vi "KB-CalRoi_Inner.vi"(10 "Inner ROI Descriptor (Inner Find Circular Edge 2)":T2={"Global Rectangle"=[775, 498, 995, 717], "Contours"=[{"ID"=enum."External", "Type"=7, "Coordinates"=[884, 607, 51, 109, 0, 0]}]} {"Contours"."Type" items=["No Selection", "Point", "Line", "Rectangle", "Oval", "Polygon", "Freehand Region", "Annulus", "Unused2", "Unused3", "Broken Line", "Freehand Line", "Rotated Rectangle"]}, 11 "Fitted Circle (Otter-Find Circular Edge)":T4 {"Average SNR (dB)" format="%.2f"; "Average Strength" format="%.2f"; "Roundness (Real-World)" format="%.2f"; "Radius (Real-World)" format="%.2f"; "Center (Real-World)"."Y" format="%.2f"; "Center (Real-World)"."X" format="%.2f"; "Radius (Pixels)" format="%.2f"; "Center (Pixels)"."Y" format="%.2f"; "Center (Pixels)"."X" format="%.2f"}) -> (0 "Roi":T1, 3 "New Inneer ROI":T2)   [LabVIEW 2015]
panel:
  out "Global Rectangle":i32[](array[numeric])
  out "元素":T3
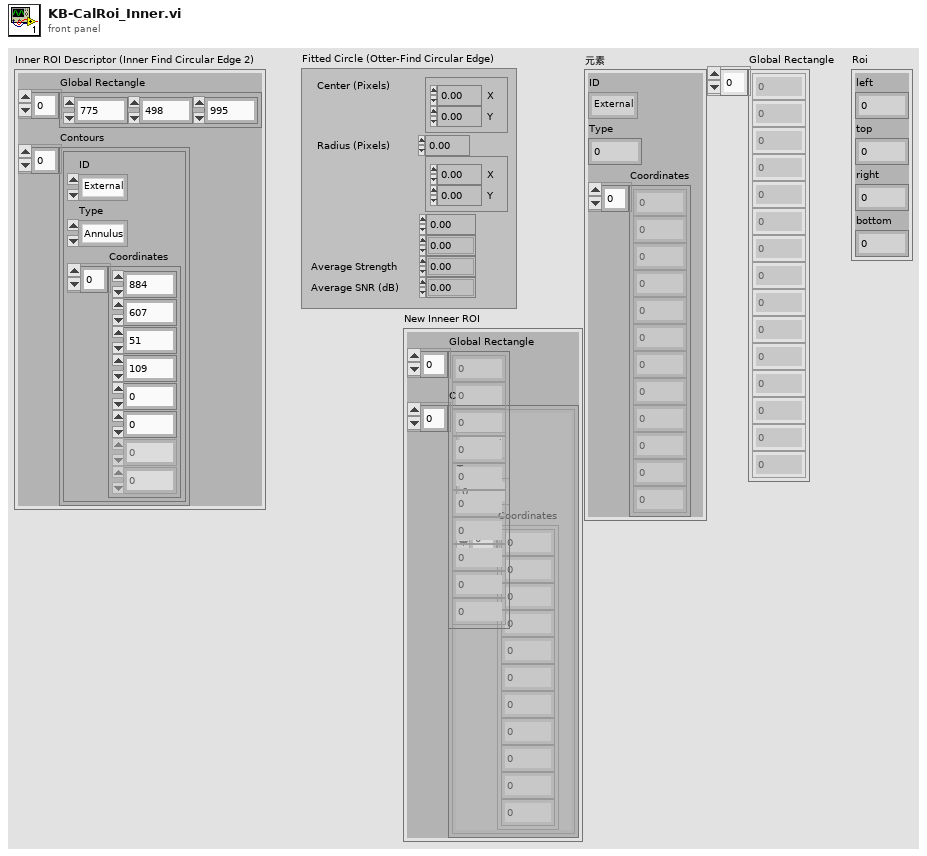
[diagram p1: front panel]
types:
  T1 = cluster{"left":dbl, "top":dbl, "right":dbl, "bottom":dbl}
  T2 = cluster{"Global Rectangle":i32[], "Contours":cluster{"ID":enum32{"External", "Internal"}, "Type":u32, "Coordinates":i32[]}[]}
  T3 = cluster{"ID":enum32{"External", "Internal"}, "Type":u32, "Coordinates":i32[]}
  T4 = cluster{"Center (Pixels)":cluster{"X":sgl, "Y":sgl}, "Radius (Pixels)":dbl, "Center (Real-World)":cluster{"X":sgl, "Y":sgl}, "Radius (Real-World)":dbl, "Roundness (Real-World)":dbl, "Average Strength":dbl, "Average SNR (dB)":dbl}
  T5 = cluster{"ID":enum32{"External", "Internal"}, "Type":u32, "Coordinates":i32[]}[]
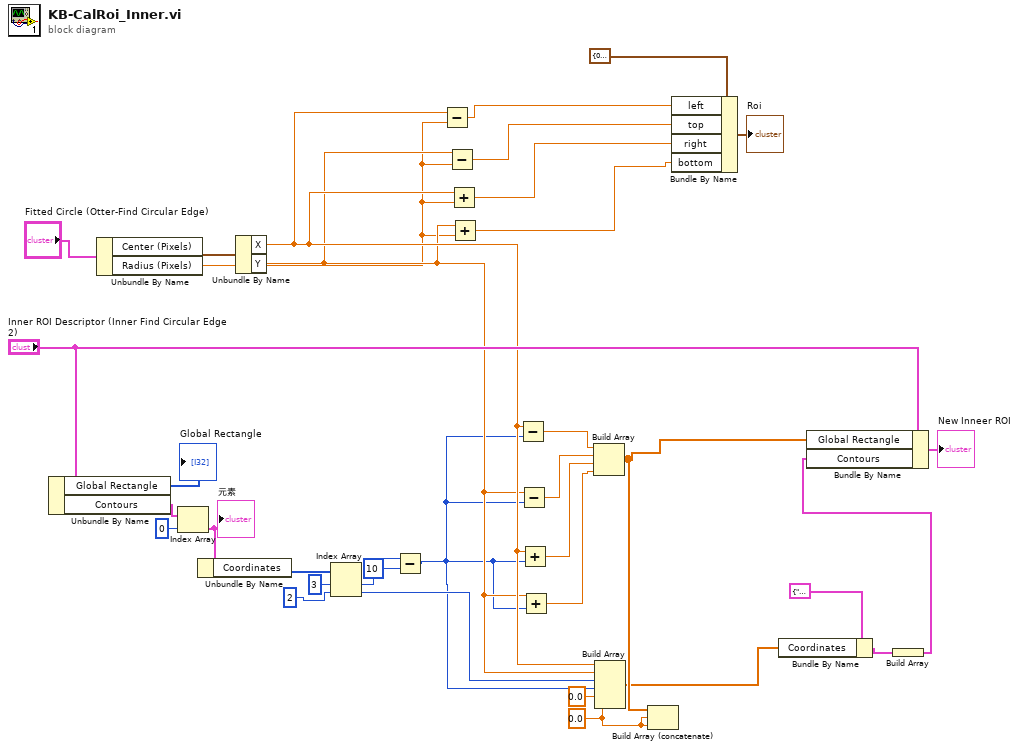
[diagram p0: block diagram]
diagram:
  w5 = sgl 0.0 ("元素")
  n1 = Unbundle By Name("Inner ROI Descriptor (Inner Find Circular Edge 2)") -> ("Global Rectangle"=→"Global Rectangle":i32[], "Contours"=w33:T5)
  n2 = Unbundle By Name("Fitted Circle (Otter-Find Circular Edge)") -> ("Center (Pixels)"=w34:cluster{"X":sgl, "Y":sgl}, "Radius (Pixels)"=w13:dbl)
  n3 = Index Array(array=w33, index=0 ("索引")) -> (element=w31:T3)
  "元素" <- w31
  n4 = Unbundle By Name(w31) -> ("Coordinates"=w30:i32[])
  n5 = Unbundle By Name(w34) -> ("X"=w15:sgl, "Y"=w14:sgl)
  n6 = Index Array(array=w30, index #1=3 ("索引"), index #2=2 ("索引")) -> (element #1=w3:i32, element #2=w20:i32)
  n7 = Subtract(x=w3, y=10) -> (x-y=w1:i32)
  n8 = Subtract(x=w15, y=w13) -> (x-y=w11:dbl)
  n9 = Subtract(x=w14, y=w13) -> (x-y=w10:dbl)
  n10 = Add(x=w15, y=w13) -> (x+y=w9:dbl)
  n11 = Add(x=w14, y=w13) -> (x+y=w8:dbl)
  n12 = Subtract(x=w15, y=w1) -> (x-y=w27:sgl)
  n13 = Subtract(x=w14, y=w1) -> (x-y=w26:sgl)
  n14 = Add(x=w15, y=w1) -> (x+y=w25:sgl)
  n15 = Add(x=w14, y=w1) -> (x+y=w24:sgl)
  n16 = Build Array(w27, w26, w25, w24) -> (w6:sgl[])
  n17 = Build Array(w15, w14, w20, w1, sgl 0.0 ("元素"), w5) -> (w4:sgl[])
  n18 = Build Array (concatenate)(w6, w5, w5) -> ()  [unwired: 1 out]
  n19 = Bundle By Name(cluster=T1 {"left"=0.0, "top"=0.0, "right"=0.0, "bottom"=0.0}, "left"=w11, "top"=w10, "right"=w9, "bottom"=w8) -> (→"Roi":T1)
  n20 = Bundle By Name(cluster=T3 {"ID"=enum."External", "Type"=7, "Coordinates"=[1645, 1058, 62, 156, 0, 0]} ("元素 2"), "Coordinates"=w4) -> (w18:T3)
  n21 = Build Array(w18) -> (w17:T5)
  n22 = Bundle By Name(cluster="Inner ROI Descriptor (Inner Find Circular Edge 2)", "Global Rectangle"=w6, "Contours"=w17) -> (→"New Inneer ROI":T2)
